vi "UDP SENDER.vi"(6 "queue":refnum<queue>, 7 "milliseconds to wait (LoopTimer)":u32, 8 "error in (no error)":errorcluster, 9 "destination adress":string, 10 "destination port":u16, 11 "UDP Network Connection in":refnum<k16>) -> (0 "error out":errorcluster)   [LabVIEW 2016]
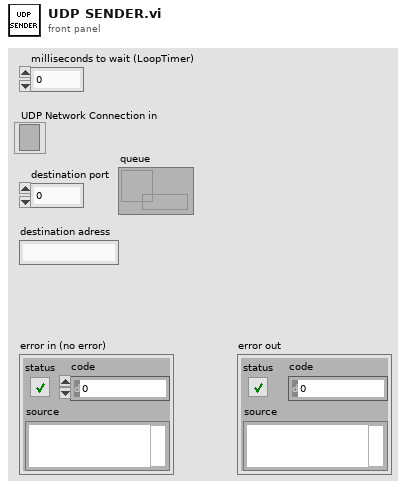
[diagram p1: front panel]
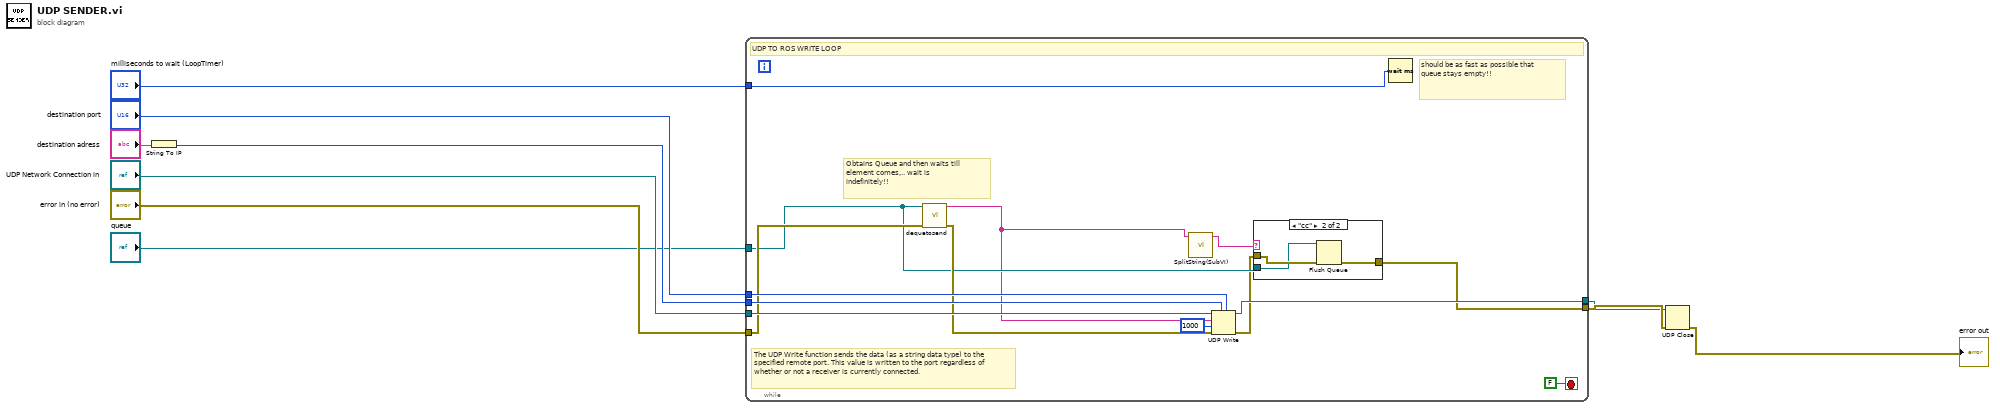
[diagram p0: block diagram]
diagram:
  n1 = String To IP(1:"destination adress") -> (0:w7:u32)
  n2 = while {
    tunnel: [w15] -> w9
    tunnel: "destination port" -> [w24]
    tunnel: w7 -> [w23]
    tunnel: "UDP Network Connection in" -> [w22]
    tunnel: "error in (no error)" -> [w19]
    tunnel: [w21] -> w8
    tunnel: "milliseconds to wait (LoopTimer)" -> [w20]
    tunnel: "queue" -> [w16]
    stop <- FALSE stop-if-true
    # "should be as fast as possible that queue stays empty!!"
    # "Obtains Queue and then waits till element comes,.. wait is indefinitely!!"
    # "The UDP Write function sends the data (as a string data type) to the specified remote port. This value is written to the port regardless of whether or not a receiver is currently connected."
    # "UDP TO ROS WRITE LOOP"
    n3 = call "dequetosend.vi"("error in (no error)"=w19, "queue"=w16) -> ("error out"=w18:errorcluster, "String to be sent"=w14:string)  [unwired: 8 in]
    n4 = call "SplitString(SubVI).vi"("data in"=w14) -> ("String 3"=w13:string)  [unwired: 9 in, 1 out]
    n5 = UDP Write(address=w23, port or service name=w24, connection ID=w22, data in=w14, 8:w18, 9:1000 ("timeout ms (25000)")) -> (error out=w12:errorcluster, 3:w21:refnum<k16>)
    n6 = case shown="\"cc\"" w13 {
      tunnel: w16 -> [_ w27]
      tunnel: w12 -> [w25 w28]
      tunnel: [w25 w26] -> w15
      frame Default {
      }
      frame "cc" {
        n7 = Flush Queue(queue=w27, error in (no error)=w28) -> (error out=w26:errorcluster)  [unwired: 2 out]
      }
    }
    n8 = Wait (ms)(milliseconds to wait=w20) -> ()  [unwired: 1 out]
  }
  n9 = UDP Close(connection ID=w8, 8:w9) -> (error out=→"error out":errorcluster)  [unwired: 1 out]
